vi "TA_Plot_SelectedSpectra.vi"(8 "Selected Time (ps)":dbl[](array[numeric])=[0.324, 0.47, 0.67, 2.02, 5.03, 32.2, 100.0, 220.0, 440.0, 1000.0], 9 "TA Data":T1={"DeltaA (mOD)"=array214x154[32956 elements], "Wavelength (nm)"=[410.231567, 411.880432, 413.529175, 415.177826, 416.826385, 418.474854, 420.123199, 421.771484, 423.419617, 425.067688, 426.715637, 428.363495, 430.01123, 431.658905, 433.306458, 434.953888, 436.601227, 438.248474, 439.89563, 441.542633, 443.189575, 444.836365, 446.483124, 448.1297, 449.776215, 451.422607, 453.068909, 454.715118, 456.361176, 458.007111, 459.653015, 461.298798, 462.944397, 464.589966, 466.235382, 467.880707, 469.52594, 471.171021, 472.815979, 474.460876, 476.105682, 477.750305, 479.394836, 481.039276, 482.683624, 484.327789, 485.971893, 487.615875, 489.259766, 490.903503, 492.54715, 494.190674, 495.834076, 497.477386, 499.120544, 500.763611, 502.406555, 504.049408, 505.692108, 507.334686, 508.977173, 510.619537, 512.261719, 513.90387, 515.545898, 517.187805, 518.82959, 520.471191, 522.112732, 523.754089, 525.395447, 527.036499, 528.677612, 530.318481, 531.959351, 533.599976, 535.24054, 536.88092, 538.521301, 540.161438, 541.801453, 543.441406, 545.081238, 546.720886, 548.360535, 549.999878, 551.639221, 553.278442, 554.917358, 556.556274, 558.195129, 559.833862, 561.472412, 563.110779, 564.749023, 566.387207, 568.025208, 569.663025, 571.300842, 572.938477, 574.575989, 576.213379, 577.850586, 579.487732, 581.124634, 582.761414, 584.398193, 586.03479, 587.671265, 589.307495, 590.943726, 592.579712, 594.215637, 595.851318, 597.487, 599.122498, 600.757874, 602.393066, 604.028259, 605.663208, 607.297913, 608.932617, 610.567078, 612.201538, 613.835815, 615.46991, 617.103943, 618.737793, 620.37146, 622.004944, 623.638428, 625.271667, 626.904846, 628.537781, 630.170715, 631.803406, 633.435974, 635.06842, 636.700623, 638.332764, 639.964783, 641.596619, 643.228333, 644.859924, 646.491272, 648.12262, 649.753662, 651.384644, 653.015442, 654.646179, 656.276672, 657.907104, 659.537292, 661.167419, 662.797302, 664.427124, 666.056702, 667.686218, 669.315552, 670.944763, 672.573792, 674.202759, 675.831421, 677.460022, 679.08844, 680.716736, 682.344849, 683.972839, 685.600708, 687.228333, 688.855896, 690.483215, 692.110413, 693.737488, 695.364319, 696.991028, 698.617676, 700.24408, 701.870361, 703.49646, 705.122375, 706.74823, 708.373779, 709.999268, 711.624634, 713.249817, 714.874817, 716.499634, 718.124329, 719.74884, 721.37323, 722.997375, 724.62146, 726.2453, 727.86908, 729.492615, 731.116028, 732.739197, 734.362244, 735.985168, 737.60791, 739.230469, 740.852905, 742.475098, 744.097229, 745.719177, 747.34082, 748.962402, 750.583801, 752.205078, 753.826172, 755.447083, 757.06781, 758.688416], "Time (ps)"=[-8.76278115, -7.76208066, -6.76138017, -5.76067968, -4.78666453, -3.78596404, -2.78526355, -1.78456306, -0.783862574, -0.717149208, -0.677121189, -0.623750496, -0.583722476, -0.530351783, -0.476981091, -0.436953071, -0.383582378, -0.330211685, -0.276840993, -0.236812973, -0.18344228, -0.130071587, -0.0767008946, -0.0366728746, 0.0166978184, 0.0700685114, 0.123439204, 0.163467224, 0.216837916, 0.270208609, 0.323579302, 0.363607321, 0.430320687, 0.470348707, 0.5237194, 0.563747419, 0.617118112, 0.670488805, 0.723859498, 0.763887517, 0.81725821, 0.870628903, 0.923999596, 0.964027615, 1.03074098, 1.070769, 1.12413969, 1.16416771, 1.21753841, 1.33762247, 1.41767851, 1.53776257, 1.61781861, 1.73790267, 1.8179587, 1.93804276, 2.0180988, 2.13818286, 2.2182389, 2.418379, 2.6185191, 2.83200187, 3.03214197, 3.23228206, 3.43242216, 3.61921959, 3.83270236, 4.01949978, 4.21963988, 4.43312265, 4.63326275, 4.82006018, 5.03354295, 5.22034037, 5.71401928, 6.22104086, 6.71471977, 7.22174135, 7.71542026, 8.22244184, 8.71612075, 9.22314233, 9.71682124, 10.2238428, 11.2245433, 12.2252438, 13.2259443, 14.2133021, 15.2140026, 16.2147031, 17.2287462, 18.2294467, 19.2301472, 20.2308477, 22.218906, 24.220307, 26.221708, 28.2364516, 30.2245099, 32.2392536, 34.2139692, 36.2287129, 38.2301139, 40.2181722, 42.2195731, 44.2343168, 46.2223751, 48.2371188, 50.2251771, 55.2153368, 60.2188393, 65.2223418, 70.2258442, 75.216004, 80.2195064, 85.2230089, 90.2131687, 95.2166711, 100.220174, 110.213836, 120.220841, 130.214503, 140.221508, 150.21517, 160.222175, 170.215837, 180.222842, 190.216504, 200.223509, 220.210834, 240.224844, 260.212168, 280.226178, 300.213502, 320.200827, 340.201494, 360.215504, 380.216171, 400.216838, 420.204162, 440.218172, 460.205497, 480.206164, 500.206831, 550.201827, 600.210167, 650.205163, 700.20016, 750.208499, 800.203495, 850.211834, 900.206831, 950.201827, 1000.21017], "Size of DeltaA"=[], "Size of Wavelength"=0, "Size of Time"=0}) -> (2 "TA Selected Spectra":cluster{"Array":dbl[], "Array 2":dbl[]}[](graph), 3 "Selected Spectra":dbl[][](array[numeric]))   [LabVIEW 2025]
uses:
  TA_DATA.ctl
panel:
  out "resulting string":string
  out "Index of Selected Time":i32[](array[numeric])
  out "Actual Selected Time":dbl[](array[numeric])
  out "DeltaA for Selected Wavelength":dbl[][](array[numeric])
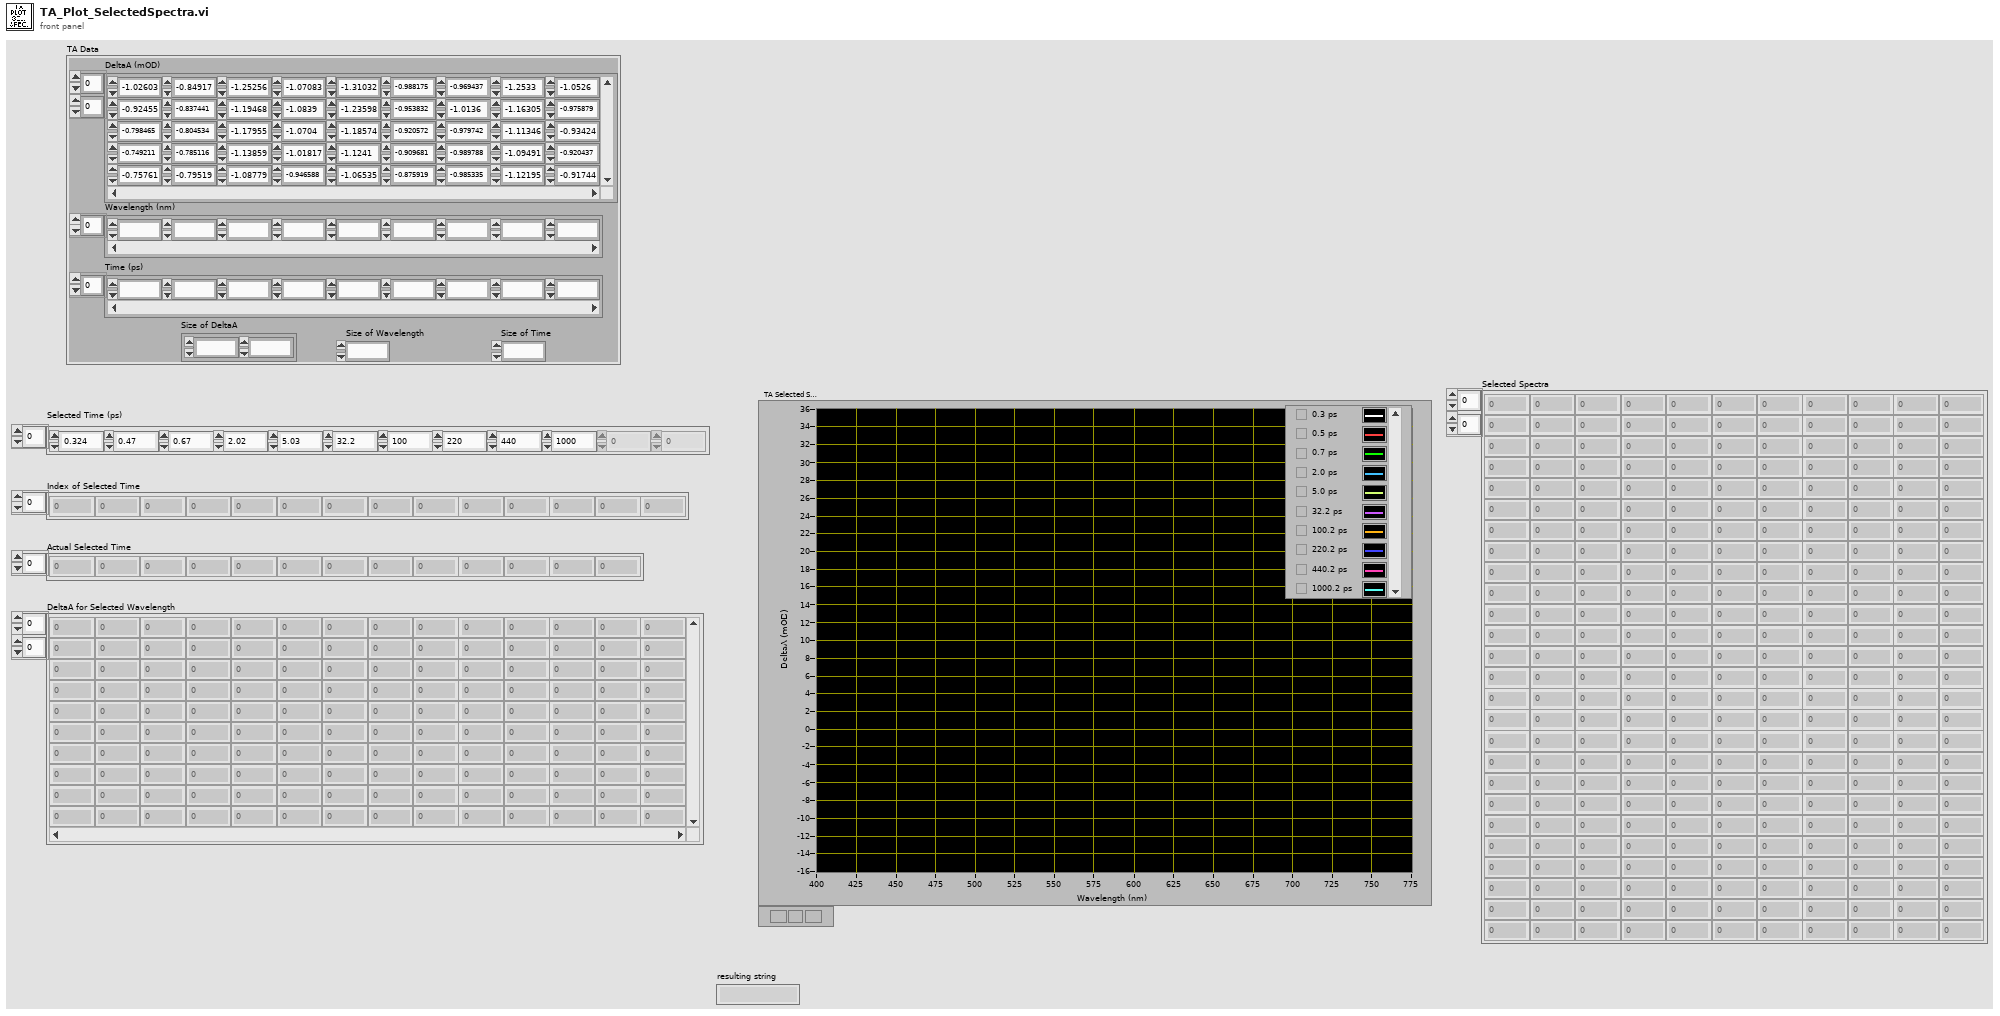
[diagram p1: front panel]
types:
  T1 = typedef "TA_DATA.ctl" = cluster{"DeltaA (mOD)":dbl[][], "Wavelength (nm)":dbl[], "Time (ps)":dbl[], "Size of DeltaA":i32[], "Size of Wavelength":i32, "Size of Time":i32}
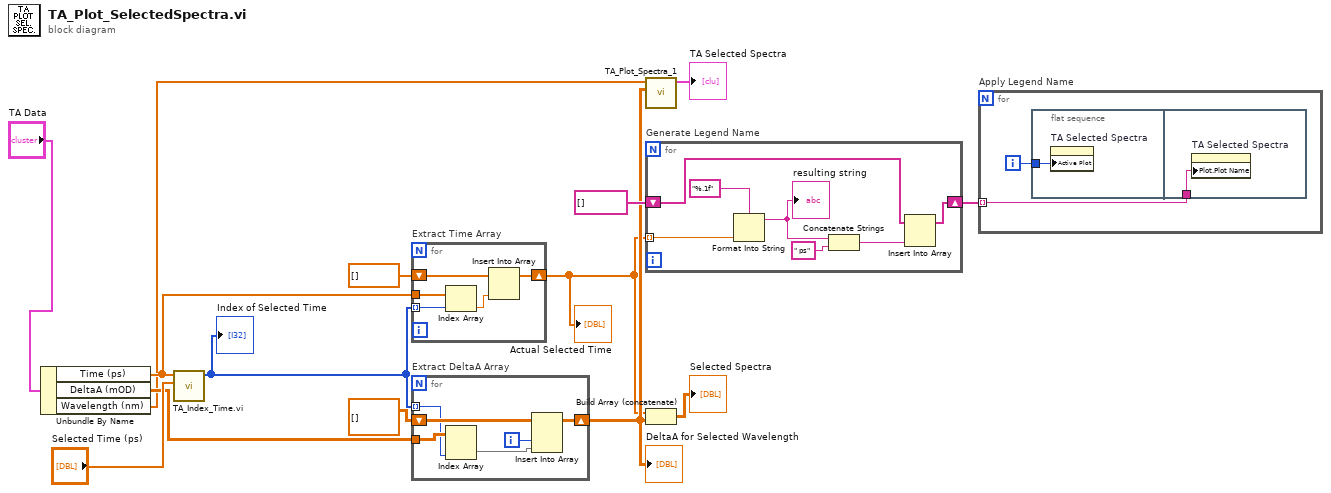
[diagram p0: block diagram]
diagram:
  n1 = Unbundle By Name("TA Data") -> ("Time (ps)"=w7:dbl[], "DeltaA (mOD)"=w6:dbl[][], "Wavelength (nm)"=w4:dbl[])
  n2 = call "TA_Index_Time.vi.vi"("Selected Time"="Selected Time (ps)", "Time (ps)"=w7) -> ("Index of Selected Time"=w8:i32[])  [unwired: 9 in]
  "Index of Selected Time" <- w8
  n3 = for "Extract Time Array" {
    shift-right: [w18] -> w2
    shift-left: dbl[] [] ("Array") -> [w17]
    tunnel: w8 -> [w19] mode=indexing
    tunnel: w7 -> [w16]
    n4 = Index Array(array=w16, index=w19) -> (element=w15:dbl)
    n5 = Insert Into Array(array=w17, new element=w15) -> (w18:dbl[])  [unwired: 1 in]
  }
  "Actual Selected Time" <- w2
  n6 = for "Extract DeltaA Array" {
    shift-right: [w24] -> w3
    shift-left: dbl[][] [] ("Array") -> [w25]
    tunnel: w8 -> [w22] mode=indexing
    tunnel: w6 -> [w23]
    i -> [w21]
    n7 = Index Array(array=w23, index (col)=w22) -> (element=w20:dbl[])  [unwired: 1 in]
    n8 = Insert Into Array(array=w25, index (col)=w21, new element=w20) -> (w24:dbl[][])  [unwired: 1 in]
  }
  "DeltaA for Selected Wavelength" <- w3
  n9 = call "TA_Plot_Spectra_1.vi"("DeltaA (mOD)"=w3, "Wavelength (nm)"=w4) -> ("TA Spectra"=→"TA Selected Spectra":cluster{"Array":dbl[], "Array 2":dbl[]}[])  [unwired: 9 in]
  n10 = for "Generate Legend Name" {
    tunnel: w2 -> [w28] mode=indexing
    shift-right: [w29] -> w11
    shift-left: string[] [] ("Array") -> [w30]
    n11 = Format Into String(format string="%.1f", w28) -> (resulting string=w26:string)  [unwired: 2 in, 1 out]
    "resulting string" <- w26
    n12 = Concatenate Strings(w26, " ps" ("string")) -> (w31:string)
    n13 = Insert Into Array(array=w30, new element=w31) -> (w29:string[])  [unwired: 1 in]
  }
  n14 = Build Array (concatenate)(w2, w3) -> (→"Selected Spectra":dbl[][])
  n15 = for "Apply Legend Name" {
    tunnel: w11 -> [w34] mode=indexing
    i -> [w33]
    n16 = flat-sequence {
      tunnel: w33 -> [w35]
      tunnel: w34 -> [w36]
      frame #0 {
        n17 = property on="TA Selected Spectra" class="XYGraph (strict)"("Active Plot"=w35) -> ()  [unwired: 2 in, 2 out]
      }
      frame #1 {
        n18 = property on="TA Selected Spectra" class="XYGraph (strict)"("Plot.Plot Name"=w36) -> ()  [unwired: 2 in, 2 out]
      }
    }
  }
